vi "AutoSelect Test Report.vi"(6 "Verbose":bool, 8 "error in (no error)":errorcluster, 9 "Test Report in":refnum<class "Test Report.lvclass">, 10 "Report Path":path) -> (0 "error out":errorcluster, 1 "Test Report out":refnum<class "Test Report.lvclass">)   [LabVIEW 2013, in "Caraya.lvlib"]
uses:
  Caraya.lvlib
  Test Report.lvclass
  Test Report.lvclass/Test Report.ctl
  Test Report.Default/Test Report.Default.lvclass
  Test Report.JUnit/Test Report.JUnit.lvclass
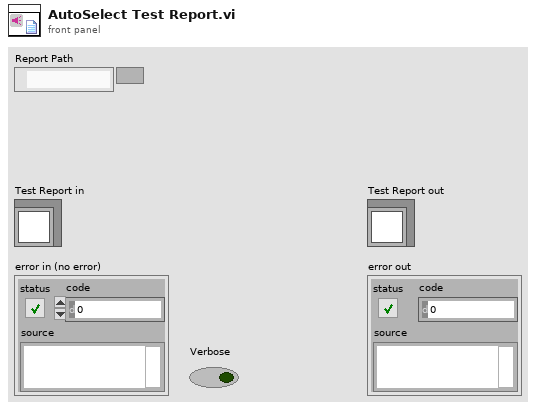
[diagram p1: front panel]
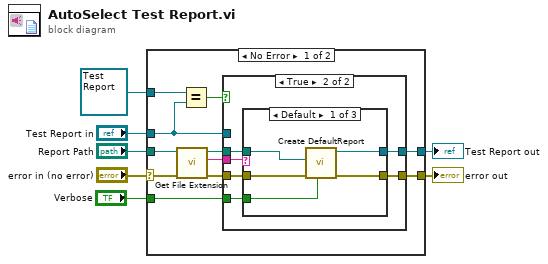
[diagram p0: block diagram]
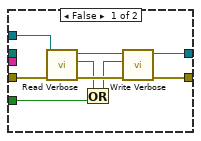
[diagram p2: hidden frame]
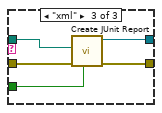
[diagram p4: hidden frame]
diagram:
  n1 = case shown="No Error" "error in (no error)" {
    selector: "error in (no error)" -> [w8 w46]
    tunnel: refnum<class "Test Report.lvclass"> refnum ("Caraya.lvlib:Test Report.lvclass") -> [w18 _]
    tunnel: [w14 w45] -> w6
    tunnel: [w13 w46] -> w5
    tunnel: "Report Path" -> [w11 _]
    tunnel: "Verbose" -> [w10 _]
    tunnel: "Test Report in" -> [w9 w45]
    frame No Error {
      n2 = call <vilib>:"Get File Extension.vi"("error in (no error)"=w8, "file"=w11) -> ("error out"=w12:errorcluster, "lowercase file extension"=w15:string, "dup file"=w16:path)  [unwired: 6 in, 1 out]
      n3 = Equal?(x=w18, y=w9) -> (x = y?=w17:bool)
      n4 = case shown="True" w17 {
        tunnel: w12 -> [w22 w33]
        tunnel: [w25 w32] -> w13
        tunnel: [w27 w31] -> w14
        tunnel: w15 -> [_ w30]
        tunnel: w16 -> [_ w29]
        tunnel: w10 -> [w21 w28]
        tunnel: w9 -> [w24 _]
        frame False {
          n5 = call "Read Verbose.vi"("error in (no error)"=w22, "Test Report in"=w24) -> ("error out"=w26:errorcluster, "Verbose"=w20:bool, "Test Report out"=w23:refnum<class "Test Report.lvclass">)  [unwired: 7 in]
          n6 = Or(x=w20, y=w21) -> (x .or. y?=w19:bool)
          n7 = call "Write Verbose.vi"("error in (no error)"=w26, "Verbose"=w19, "Test Report in"=w23) -> ("error out"=w25:errorcluster, "Test Report out"=w27:refnum<class "Test Report.lvclass">)  [unwired: 7 in]
        }
        frame True {
          n8 = case shown="Default" w30 {
            tunnel: w33 -> [w38 w39 w44]
            tunnel: [w37 w39 w43] -> w32
            tunnel: [w36 _ w42] -> w31
            tunnel: w29 -> [w35 _ w41]
            tunnel: w28 -> [w34 _ w40]
            frame Default {
              n9 = call "Create DefaultReport.vi"("Verbose"=w34, "error in (no error)"=w38, "Report Path"=w35) -> ("error out"=w37:errorcluster, "Test Report.Default out"=w36:refnum<class "Test Report.Default.lvclass">)  [unwired: 7 in]
            }
            frame "" {
            }
            frame "xml" {
              n10 = call "Create JUnit Report.vi"("Verbose"=w40, "error in (no error)"=w44, "Report Path"=w41) -> ("error out"=w43:errorcluster, "Test Report.JUnit out"=w42:refnum<class "Test Report.JUnit.lvclass">)  [unwired: 7 in]
            }
          }
        }
      }
    }
    frame Error {
    }
  }
  "Test Report out" <- w6
  "error out" <- w5
